vi "aquireAccelerationData.vi"(8 "ErrorIn":errorcluster, 11 "QueuesIn":T1) -> (0 "ErrorOut":errorcluster, 3 "QueuesOut":T1)   [LabVIEW 2019]
uses:
  utilities/AQueues.ctl
  AmasterVIs/ACommand.ctl
  analyzeAccelerationDataVIs/AccelerationDataFrames.ctl
  analyzeAccelerationDataVIs/AnalyzedVibrationsData.ctl
  analyzeAccelerationDataVIs/calculateFaultIndicatorsVIs/FaultDetections.ctl
  analyzeAccelerationDataVIs/calculateFaultIndicatorsVIs/ParameterFaultDetection.ctl
  analyzeAccelerationDataVIs/calculateFaultIndicatorsVIs/FaultParameter.ctl
  analyzeAccelerationDataVIs/calculateFaultIndicatorsVIs/FrequencyFaultDetection.ctl
  analyzeAccelerationDataVIs/calculateFaultIndicatorsVIs/OrdersFaultDetection.ctl
  TDMSmanagerVIs/TDMSAnalyzerData.ctl
  TDMSmanagerVIs/TDMSAnalyzerDataType.ctl
  aquireAccelerationDataVIs/aquireAccelerationDataState.ctl
  AmasterVIs/AThreads.ctl
  aquireAccelerationDataVIs/Operation.ctl
  UIVIs/UIOutputFGVAction.ctl
panel:
  in  "Restart":bool
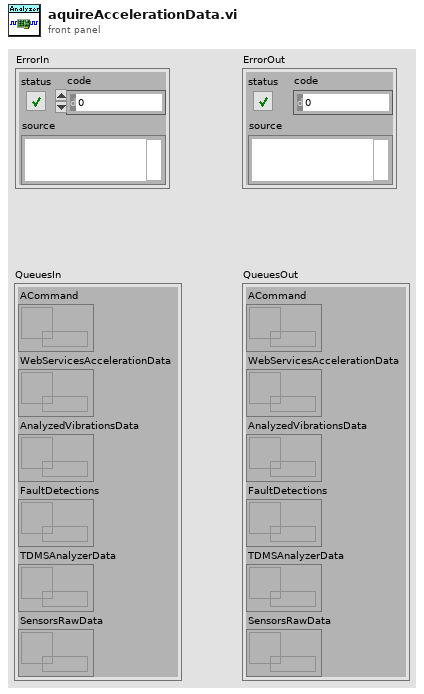
[diagram p1: front panel]
types:
  T1 = typedef "AQueues.ctl" = cluster{"ACommand":refnum<queue>, "WebServicesAccelerationData":refnum<queue>, "AnalyzedVibrationsData":refnum<queue>, "FaultDetections":refnum<queue>, "TDMSAnalyzerData":refnum<queue>, "SensorsRawData":refnum<queue>}
  T2 = typedef "aquireAccelerationDataState.ctl" = enum16{"Idle", "Connect", "AquireData", "EndConnection"}
  T3 = typedef "AThreads.ctl" = enum16{"UI", "analyzeAccelerationData", "aquireAccelerationData", "communicateWebServices", "TDMSmanager", "aquireTachoSignal"}
  T4 = typedef "ACommand.ctl" = enum16{"None", "Start", "Stop", "Restart", "SendFilesData", "DeleteAllData"}
  T5 = typedef "Operation.ctl" = enum16{"Initialize Connection", "Read Data", "Close Connection", "Calculate Data To g"}
  T6 = typedef "UIOutputFGVAction.ctl" = enum16{"Read", "Write", "CheckUpdate"}
  T7 = typedef "UIOutput.ctl" = cluster{"Aquiring data":bool, "AnalyzerError":errorcluster, "FIFO overflow":bool, "Analyzing data":bool}
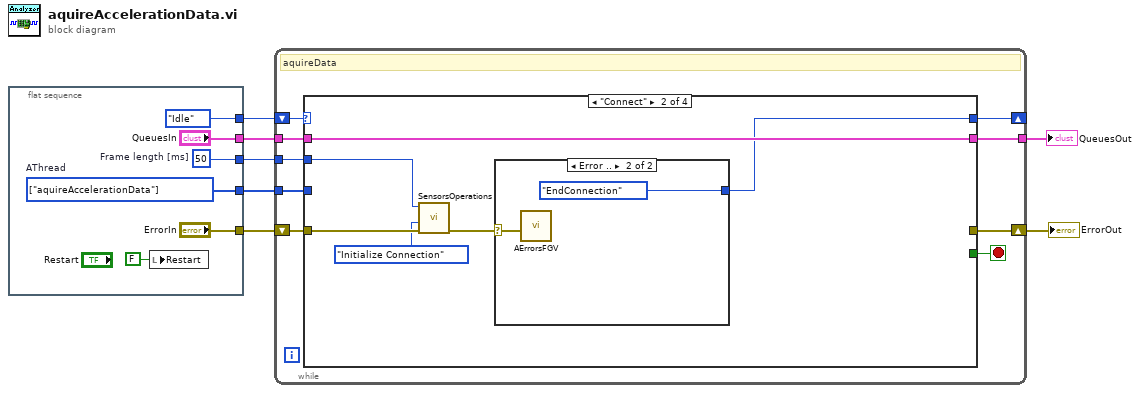
[diagram p0: block diagram]
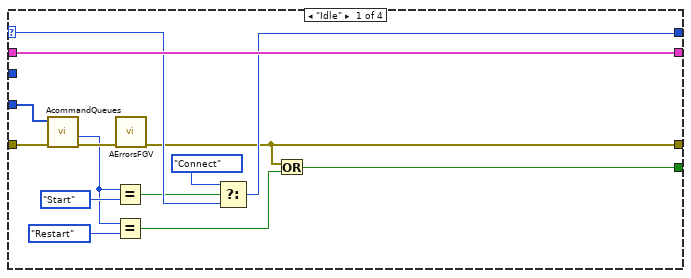
[diagram p2: hidden frame]
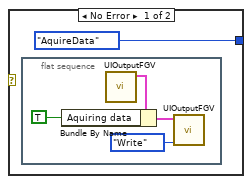
[diagram p3: hidden frame]
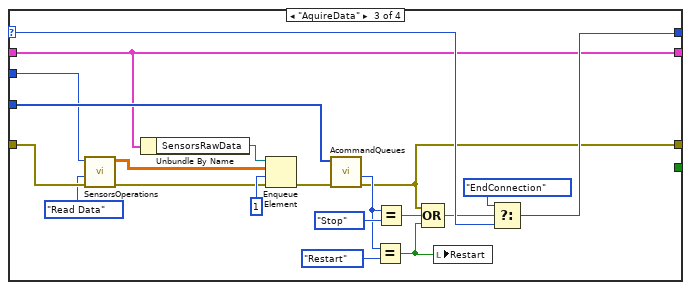
[diagram p4: hidden frame]
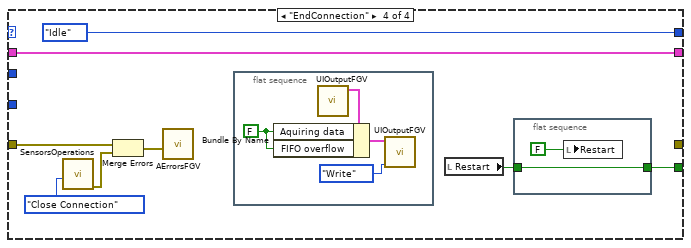
[diagram p5: hidden frame]
diagram:
  n1 = flat-sequence {
    tunnel: [aquireAccelerationDataState."Idle" ("aquireAccelerationDataState")] -> w7
    tunnel: ["QueuesIn"] -> w6
    tunnel: ["ErrorIn"] -> w5
    tunnel: [w9] -> w2
    tunnel: [w8] -> w1
    frame #0 {
      w8 = i64 50  # Frame length [ms]
      w9 = T3[] [enum."aquireAccelerationData"] items=["UI", "analyzeAccelerationData", "aquireAccelerationData", "communicateWebServices", "TDMSmanager", "aquireTachoSignal"]  # AThread
      n2 = local write "Restart"(FALSE ("Restart")) -> ()
    }
  }
  n3 = while {
    shift-right: [w18] -> _
    shift-left: w7 -> [w22]
    tunnel: w6 -> [w21]
    shift-right: [w17] -> w4
    shift-left: w5 -> [w20]
    tunnel: [w16] -> w3
    tunnel: w2 -> [w15]
    tunnel: w1 -> [w14]
    stop <- w19 stop-if-true
    # "aquireData"
    n4 = case shown="\"Connect\"" w22 {
      selector: w22 -> [w35 _ w68 _]
      tunnel: [w36 w42 w66 w77] -> w16
      tunnel: w21 -> [w36 w42 w66 w77]
      tunnel: w20 -> [w27 w40 w57 w70]
      tunnel: [w28 _ w50 _] -> w17
      tunnel: [w23 _ _ w75] -> w19
      tunnel: [w33 w41 w69 aquireAccelerationDataState."Idle" ("aquireAccelerationDataState")] -> w18
      tunnel: w15 -> [w25 _ w67 _]
      tunnel: w14 -> [_ w39 w56 _]
      frame "Idle" {
        n5 = call "AcommandQueues.vi"("ErrorIn"=w27, "AThreads"=w25) -> ("ErrorOut"=w26:errorcluster, "ACommandOut"=w24:T4)  [unwired: 8 in]
        n6 = Equal?(x=w24, y=ACommand."Start") -> (x = y?=w30:bool)
        n7 = Equal?(x=w24, y=ACommand."Restart") -> (x = y?=w29:bool)
        n8 = call "AErrorsFGV.vi"("CriticalErrorIn"=w26) -> ("CriticalErrorOut"=w28:errorcluster)  [unwired: 7 in, 3 out]
        n9 = Select(t=aquireAccelerationDataState."Connect", s=w30, f=w35) -> (s? t:f=w33:T2)
        n10 = Or(x=w28, y=w29) -> (x .or. y?=w23:bool)
      }
      frame "Connect" {
        n11 = call "SensorsOperations.vi"("ErrorIn"=w40, "Operation"=Operation."Initialize Connection", "frame length ms"=w39) -> ("ErrorOut"=w37:errorcluster)  [unwired: 5 in, 3 out]
        n12 = case shown="Error .." w37 {
          selector: w37 -> [_ w48]
          tunnel: [aquireAccelerationDataState."AquireData" ("aquireAccelerationDataState") aquireAccelerationDataState."EndConnection" ("aquireAccelerationDataState")] -> w41
          frame No Error {
            n13 = flat-sequence {
              frame #0 {
                n14 = call "UIOutputFGV.vi"() -> ("UIOutputOut"=w47:T7)  [unwired: 10 in, 1 out]
                n15 = Bundle By Name(cluster=w47, "Aquiring data"=TRUE) -> (w45:T7)
                n16 = call "UIOutputFGV.vi"("FGVAction (Read)"=UIOutputFGVAction."Write", "UIOutputIn"=w45) -> ()  [unwired: 8 in, 2 out]
              }
            }
          }
          frame Error {
            n17 = call "AErrorsFGV.vi"("InternalErrorIn"=w48) -> ()  [unwired: 7 in, 4 out]
          }
        }
      }
      frame "AquireData" {
        n18 = call "SensorsOperations.vi"("ErrorIn"=w57, "Operation"=Operation."Read Data", "frame length ms"=w56) -> ("ErrorOut"=w54:errorcluster, "RawAccelerationData Out"=w51:dbl[][])  [unwired: 5 in, 2 out]
        n19 = Unbundle By Name(w66) -> ("SensorsRawData"=w53:refnum<queue>)
        n20 = Enqueue Element(queue=w53, element=w51, timeout in ms (-1)=1, error in (no error)=w54) -> (error out=w52:errorcluster)  [unwired: 2 out]
        n21 = call "AcommandQueues.vi"("ErrorIn"=w52, "AThreads"=w67) -> ("ErrorOut"=w50:errorcluster, "ACommandOut"=w58:T4)  [unwired: 8 in]
        n22 = Equal?(x=w58, y=ACommand."Restart") -> (x = y?=w59:bool)
        n23 = Equal?(x=w58, y=ACommand."Stop") -> (x = y?=w60:bool)
        n24 = Compound Arithmetic op=OR(w50, w60, w59) -> (w65:bool)
        n25 = local write "Restart"(w59) -> ()
        n26 = Select(t=aquireAccelerationDataState."EndConnection", s=w65, f=w68) -> (s? t:f=w69:T2)
      }
      frame "EndConnection" {
        n27 = call "SensorsOperations.vi"("Operation"=Operation."Close Connection") -> ("ErrorOut"=w72:errorcluster)  [unwired: 7 in, 3 out]
        n28 = Merge Errors(w70, w72) -> (w71:errorcluster)
        n29 = call "AErrorsFGV.vi"("InternalErrorIn"=w71) -> ()  [unwired: 7 in, 4 out]
        n30 = flat-sequence {
          frame #0 {
            w80 = FALSE ("Aquiring data")
            n31 = call "UIOutputFGV.vi"() -> ("UIOutputOut"=w83:T7)  [unwired: 10 in, 1 out]
            n32 = Bundle By Name(cluster=w83, "Aquiring data"=w80, "FIFO overflow"=w80) -> (w82:T7)
            n33 = call "UIOutputFGV.vi"("FGVAction (Read)"=UIOutputFGVAction."Write", "UIOutputIn"=w82) -> ()  [unwired: 8 in, 2 out]
          }
        }
        n34 = local read "Restart"() -> (w74:bool)
        n35 = flat-sequence {
          tunnel: [w78] -> w75
          tunnel: w74 -> [w78]
          frame #0 {
            n36 = local write "Restart"(FALSE ("Restart")) -> ()
          }
        }
      }
    }
  }
  "ErrorOut" <- w4
  "QueuesOut" <- w3
